vi "Init_Test.vi"(8 "error in (no error)":errorcluster caption="entrée d'erreur (pas d'erreur)", 11 "Print_Label en entrée":refnum<class "P2056_Wait_Start.lvclass">) -> (0 "error out":errorcluster caption="sortie d'erreur", 3 "Print_Label en sortie":refnum<class "P2056_Wait_Start.lvclass">)   [LabVIEW 2020, in "Library Test.lvlib" / "P2056_Wait_Start.lvclass"]
uses:
  P2056_Wait_Start.lvclass
  C:/Users/ngarcin/OneDrive - Altyor/Standard TB/Class/Test/Test (Default)/Test (Default).lvclass
  Commun VI/TypeDef/Commande Test/Commande Type Test.ctl
  P2056_Send_Command_UART/P2056_Send_Command_UART.lvclass
  P2056_Wait_Start.lvclass/P2056_Wait_Start.ctl
  Commun VI/Library Commun.lvlib
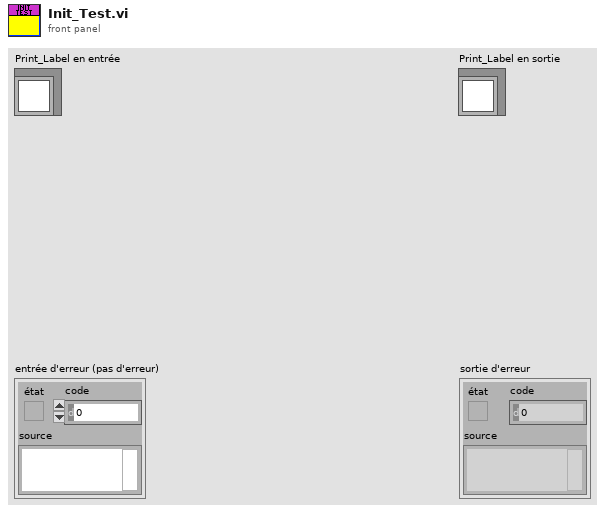
[diagram p1: front panel]
types:
  T1 = typedef "Library Commun.lvlib/Commande Type Test.ctl" = enum16{"Function", "Test", "Calculation"}
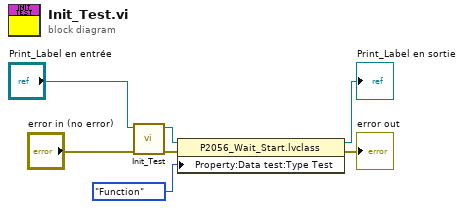
[diagram p0: block diagram]
diagram:
  n1 = call-parent "Init_Test.vi"("error in (no error)"="error in (no error)", "Print_Label en entrée"="Print_Label en entrée") -> ("error out"=w2:errorcluster, "Print_Label en sortie"=w5:refnum<class "P2056_Wait_Start.lvclass">)  [unwired: 8 in]
  n2 = property class="P2056_Wait_Start.lvclass"(reference=w5, error in=w2, "Property:Data test:Type Test"=Commande_Type_Test."Function" ("Type Test")) -> (reference out=→"Print_Label en sortie":refnum<class "P2056_Wait_Start.lvclass">, error out=→"error out":errorcluster)
